vi "PreLoading.vi"(4 "Voltage":dbl=5.0 format="%#_13g", 5 "Direction":T1, 6 "target pressure [MPa]":dbl=3.0 format="%#_13g", 7 "init":bool, 8 "error in (no error)":errorcluster, 11 "Stand in":refnum<class "Stand.lvclass">) -> (0 "error out":errorcluster, 2 "done":bool, 3 "Stand out":refnum<class "Stand.lvclass">)   [LabVIEW 2019, in "Stand.lvclass"]
uses:
  Stand.lvclass
  C:/Users/ANENKOV_V1/Desktop/src/Device_class/Device.lvclass
  TypeDef/Direction.ctl
  TypeDef/SP_TYPE.ctl
  Stand.lvclass/Stand.ctl
  AI_class/AI.lvclass/AI.ctl
  AnalogComparator_class/AnalogComparator.lvclass/AnalogComparator.ctl
  Device_class/Device.lvclass/Device.ctl
  Valve Mode.ctl
  c2c3d155-81bf-490b-b50d-397c388f1e85.vi
  AnalogComparator_class/GetStatus.vi
  Valve State Mode.vi
  Valve State Mode.vi/810e184e-eeb6-4027-a8ae-1422f3ce3d45.vi
  Valve State Mode.vi/57bd4a65-f3dc-44f5-8d68-677c2a197570.vi
  Valve State Mode.vi/03b2f9e4-fceb-4725-9b90-3fd10082a088.vi
  Valve State Mode.vi/3d0d09bd-48e8-482f-b1e2-a36b2bb65234.vi
  Valve State Mode.vi/33d3f26a-dc4a-4f56-bf0a-61d04c5d7434.vi
  Valve State Mode.vi/52af9d47-24d1-4057-80bf-8d93bfb3d17d.vi
  Valve State Mode.vi/094228cb-a119-423c-9af8-5a16f059a318.vi
  Valve State Mode.vi/bf5ad1e6-a0ae-4579-ad74-ca8f304cb7cf.vi
  Valve State Mode.vi/eb4d2b76-f0f0-4e1d-bda0-609c5f37b4e7.vi
  Const All Valve.vi
  FPGA/TypeDef/DO index.ctl
  FPGA_API_class/FPGA API.lvclass
  Device_class/Device.lvclass
  AI_class/AI.lvclass
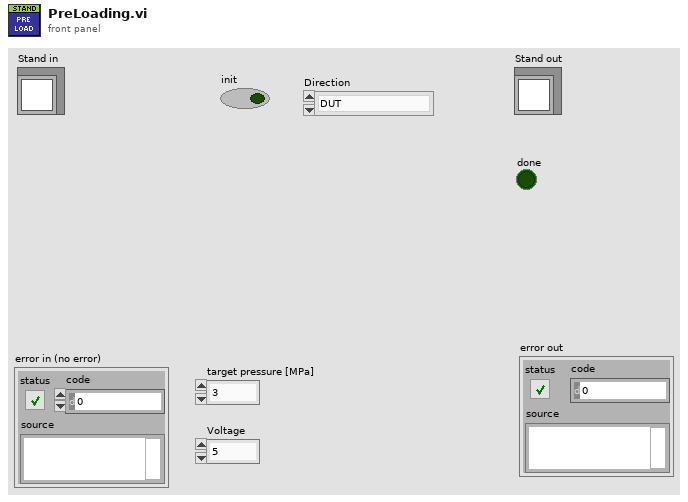
[diagram p1: front panel]
types:
  T1 = typedef "Direction.ctl" = enum8{"DUT", "Chamber"}
  T2 = typedef "SP_TYPE.ctl" = enum16{"ERROR", "ZIRO", "BASE", "SP"}
  T3 = typedef "Valve Mode.ctl" = enum16{"Filling DUT", "Filling Chamber", "Pump Pressure DUT", "Pump Pressure Chamber", "Haskel Pressure DUT", "Haskel Pressure Chamber", "Slow Release DUT", "Slow Release Chamber", "Fast Release DUT", "Fast Release Chamber", "Fast Release DUT and Chamber", "Leak Pressure DUT", "Leak Pressure Chamber", "Back Pressure DUT", "Back Pressure Chamber", "Fully Closed", "Drain", "Block DUT", "Block Chamber"}
  T4 = typedef "AI_Data.ctl" = cluster{"Stat Data":T5, "OutOfRangeMax":bool, "OutOfRangeMin":bool, "HIHI":bool, "HI":bool, "LO":bool, "LOLO":bool}
  T5 = typedef "AI Statistics Data.ctl" = cluster{"raw mean":dbl, "scl mean":dbl, "raw mean 1Hz":dbl, "scl mean 1Hz":dbl}
  T6 = typedef "DO index.ctl" = u8
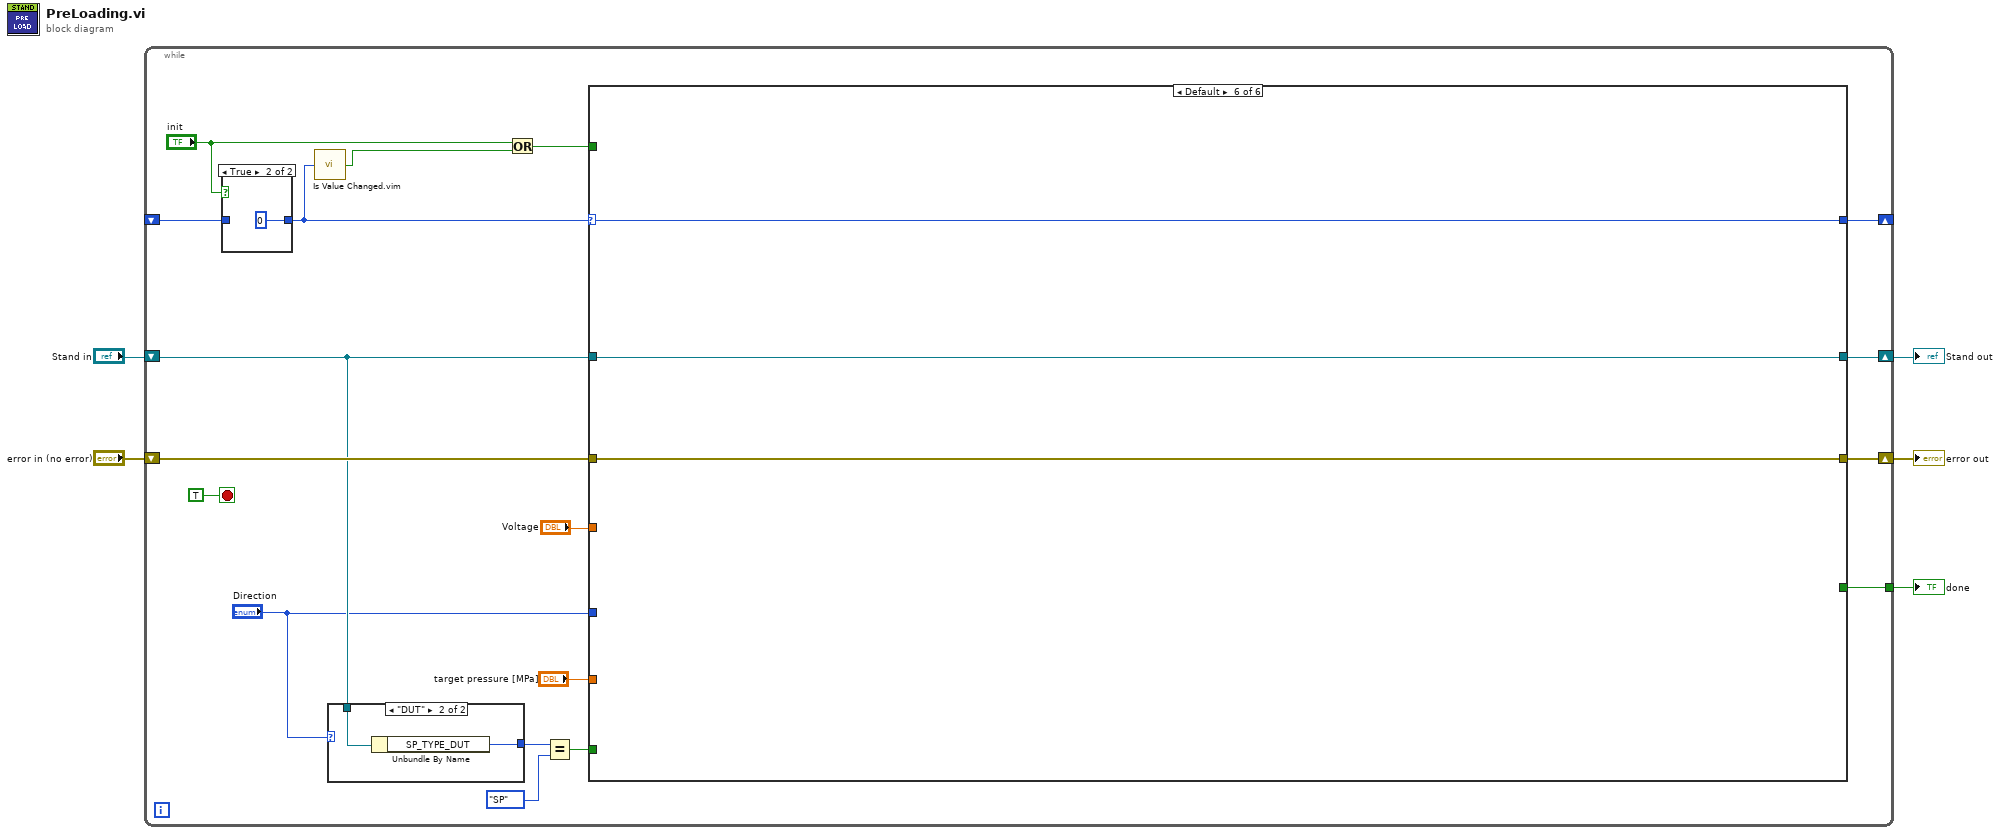
[diagram p0: block diagram]
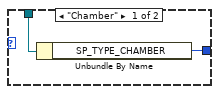
[diagram p2: hidden frame]
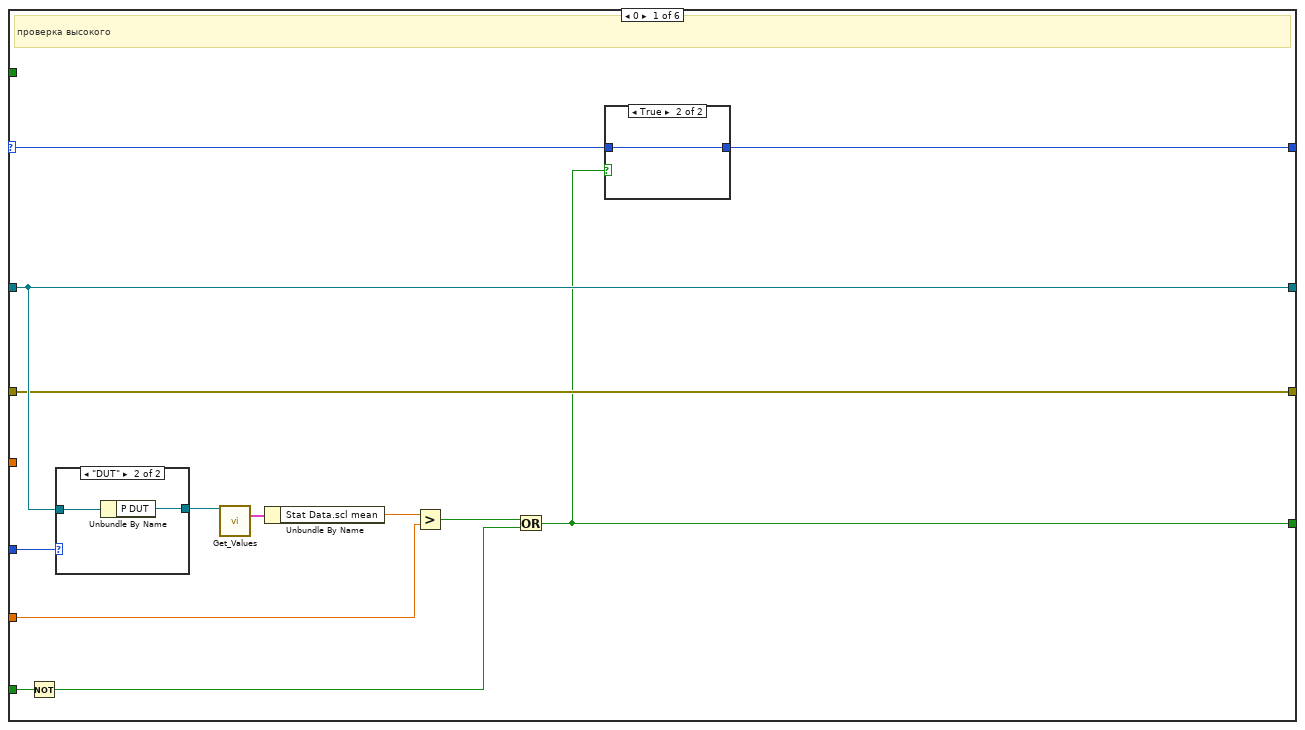
[diagram p4: hidden frame]
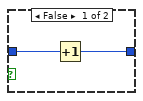
[diagram p5: hidden frame]
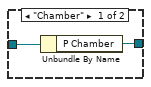
[diagram p6: hidden frame]
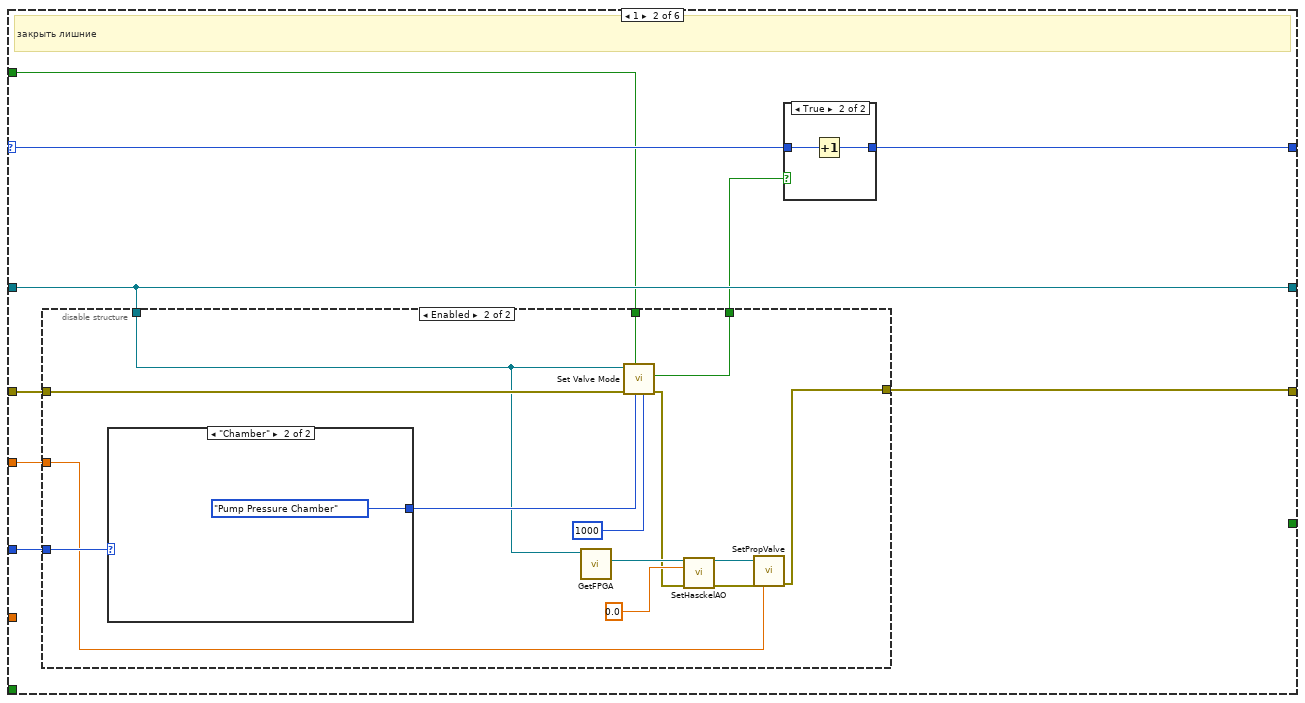
[diagram p7: hidden frame]
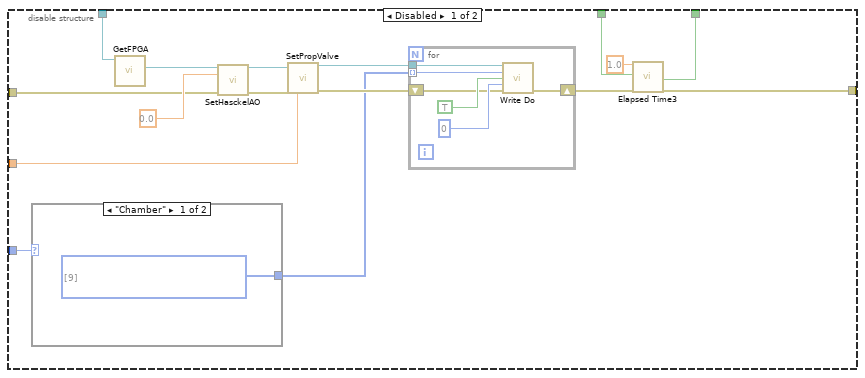
[diagram p8: hidden frame]
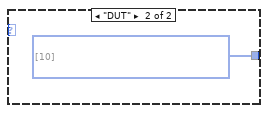
[diagram p9: hidden frame]
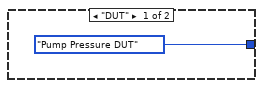
[diagram p10: hidden frame]
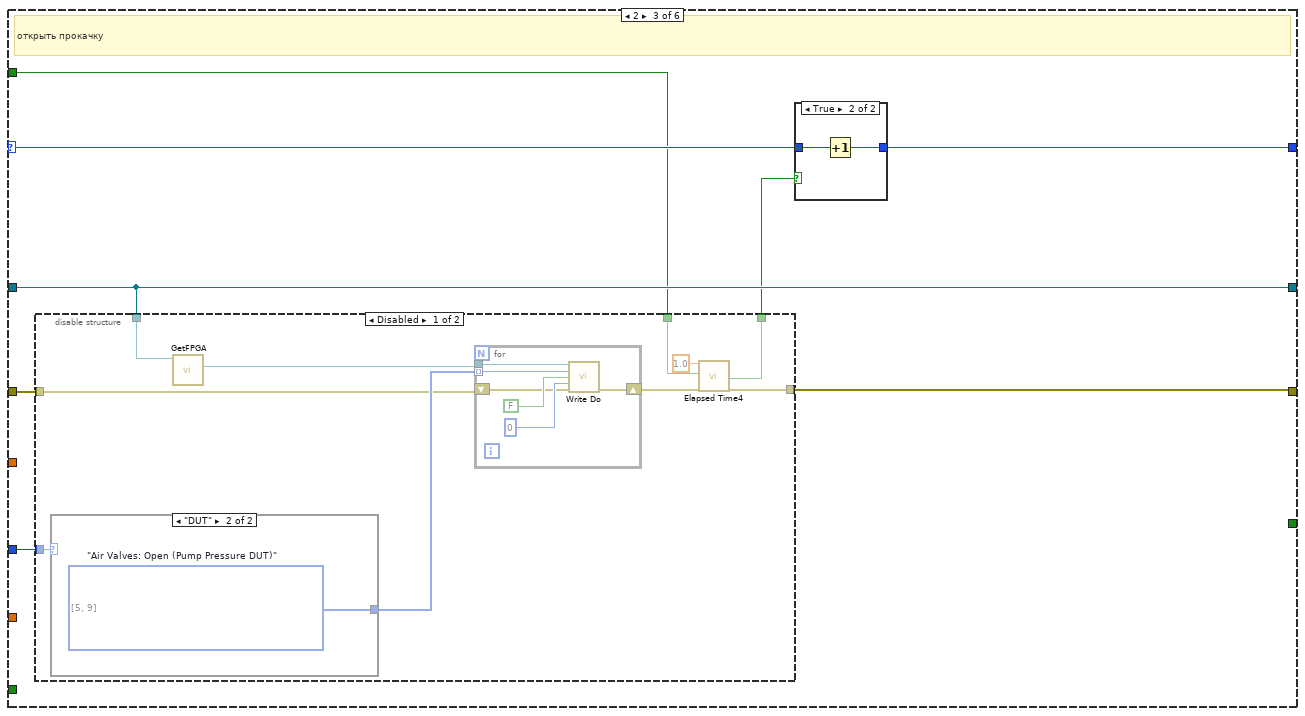
[diagram p12: hidden frame]
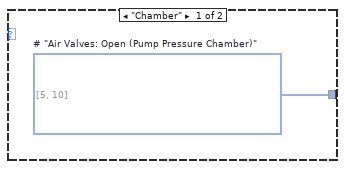
[diagram p13: hidden frame]
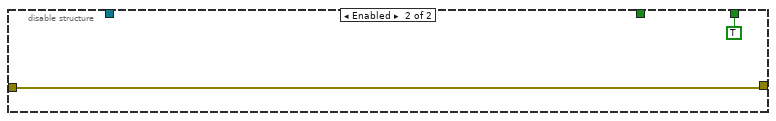
[diagram p14: hidden frame]
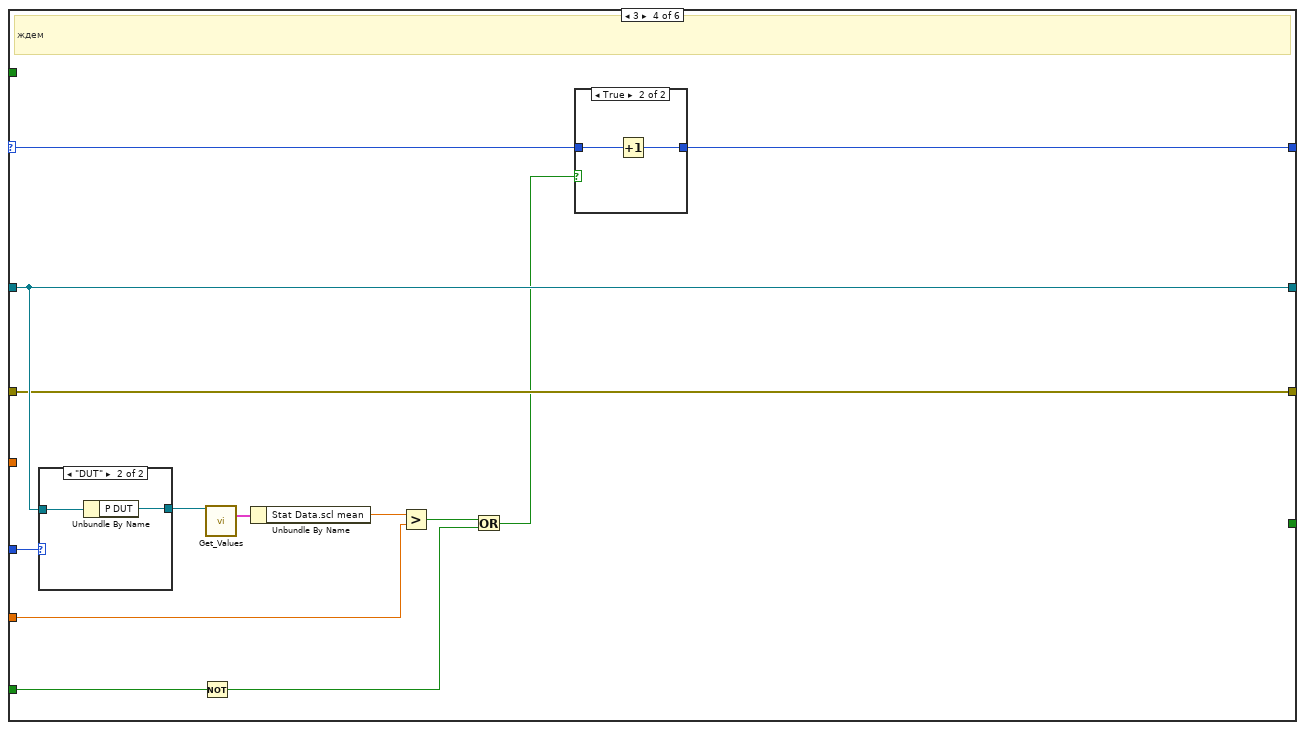
[diagram p16: hidden frame]
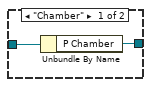
[diagram p18: hidden frame]
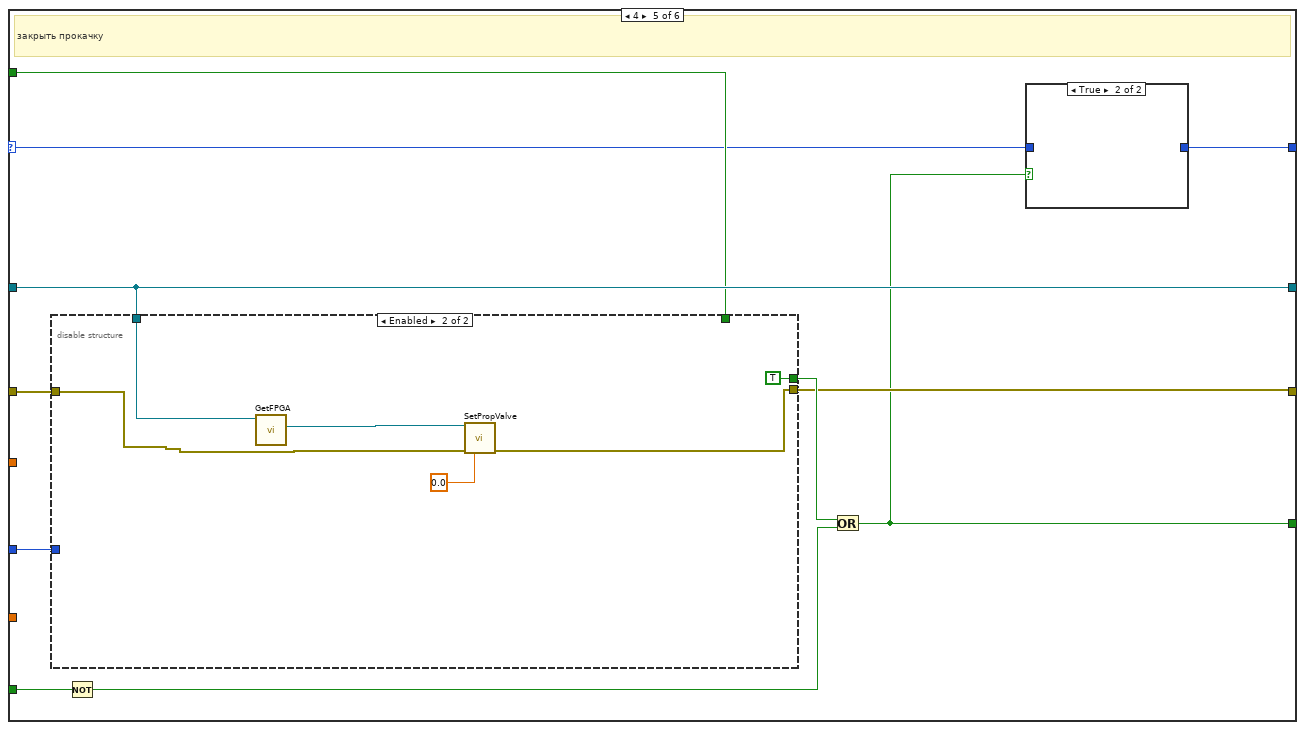
[diagram p19: hidden frame]
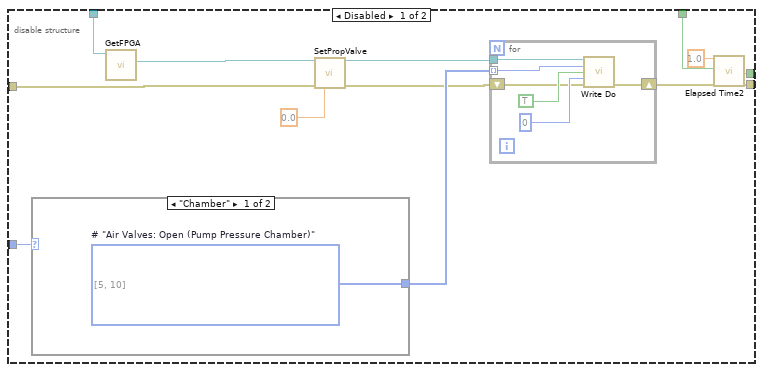
[diagram p20: hidden frame]
diagram:
  n1 = while {
    shift-right: [w21] -> _
    shift-left: _ -> [w18]
    tunnel: [w15] -> w4
    shift-right: [w14] -> w2
    shift-left: "Stand in" -> [w10]
    shift-right: [w13] -> w1
    shift-left: "error in (no error)" -> [w12]
    stop <- TRUE stop-if-true
    n2 = case shown="True" "init" {
      tunnel: w18 -> [w28 _]
      tunnel: [w28 0] -> w17
      frame False {
      }
      frame True {
      }
    }
    n3 = call "Is Value Changed.vim"("value"=w17) -> ("changed or first call?"=w22:bool)
    n4 = case shown="\"DUT\"" "Direction" {
      tunnel: w10 -> [w25 w27]
      tunnel: [w24 w26] -> w8
      frame "Chamber" {
        n5 = Unbundle By Name(w25) -> ("SP_TYPE_CHAMBER"=w24:T2)
      }
      frame "DUT" {
        n6 = Unbundle By Name(w27) -> ("SP_TYPE_DUT"=w26:T2)
      }
    }
    n7 = Or(x="init", y=w22) -> (x .or. y?=w19:bool)
    n8 = Equal?(x=w8, y=SP_TYPE."SP") -> (x = y?=w6:bool)
    n9 = case shown="Default" w17 {
      selector: w17 -> [w42 w58 w109 w145 w154 w194]
      tunnel: [w41 w57 w108 w144 w153 w194] -> w21
      tunnel: w19 -> [_ w52 w104 _ w161 _]
      tunnel: w10 -> [w34 w56 w107 w138 w163 w193]
      tunnel: "Direction" -> [w40 w53 w105 w143 w162 _]
      tunnel: "target pressure [MPa]" -> [w36 _ _ w139 _ _]
      tunnel: [w30 _ _ _ w155 _] -> w15
      tunnel: [w34 w56 w107 w138 w163 w193] -> w14
      tunnel: [w33 w50 w102 w137 w159 w192] -> w13
      tunnel: w12 -> [w33 w55 w106 w137 w158 w192]
      tunnel: "Voltage" -> [_ w54 _ _ _ _]
      tunnel: w6 -> [w32 _ _ w134 w157 _]
      frame 0 {
        # "проверка высокого"
        n10 = Not(x=w32) -> (.not. x?=w31:bool)
        n11 = case shown="\"DUT\"" w40 {
          tunnel: w34 -> [w47 w49]
          tunnel: [w46 w48] -> w37
          frame "Chamber" {
            n12 = Unbundle By Name(w47) -> ("P Chamber"=w46:refnum<class "AI.lvclass">)
          }
          frame "DUT" {
            n13 = Unbundle By Name(w49) -> ("P DUT"=w48:refnum<class "AI.lvclass">)
          }
        }
        n14 = call "Get_Values.vi"("reference in"=w37) -> ("Data"=w38:T4)  [unwired: 14 in]
        n15 = Unbundle By Name(w38) -> ("Stat Data.scl mean"=w39:dbl)
        n16 = Greater?(x=w39, y=w36) -> (0:w35:bool)
        n17 = Or(x=w35, y=w31) -> (x .or. y?=w30:bool)
        n18 = case shown="True" w30 {
          tunnel: w42 -> [w44 w45]
          tunnel: [w43 w45] -> w41
          frame False {
            n19 = Increment(x=w44) -> (x+1=w43:i32)
          }
          frame True {
          }
        }
      }
      frame 1 {
        # "закрыть лишние"
        n20 = disable-structure shown="Enabled" {
          disable-tunnel: w56 -> [w67 w86]
          disable-tunnel: w55 -> [w66 w95]
          disable-tunnel: w54 -> [w65 w85]
          disable-tunnel: w53 -> [w64 w92]
          disable-tunnel: w52 -> [w62 w96]
          disable-tunnel: [w60 w94] -> w51
          disable-tunnel: [w59 w83] -> w50
          frame Disabled {
            n21 = case shown="\"Chamber\"" w64 {
              tunnel: [w81 w82] -> w68
              frame "Chamber" {
                w81 = T6[] [9] items=["DO 0 [KP1] [M12]", "DO 1 [ON KP2] [M21]", "DO 2 [ON KP3] [M24]", "DO 3 [WATER Y18.1 [DO3]]", "DO 4 [WATER Y18.2 [DO4]]", "DO 5 [KP6 Y29.1 33.7]", "DO 6 [KP7 Y29.2 33.8]", "DO 7 [KP8 Y29.3 33.9]", "DO 8 [KP9 Y29.4  33.12]", "DO 9 [KP10 Y29.5 33.1]", "DO 10 [KP11 Y29.6 33.2]", "DO 11 [KP12 Y29.7  33.13]", "DO 12 [KP13 Y29.8  33.11]", "DO 13 [KP14 Y29.9 33.10]", "DO 14 [KP15 Y29.10  33.6]", "DO 15 [KP16 Y29.11  33.5]", "DO 16 [KP17 Y29.12  33.4]", "DO 17 [KP18 Y29.13 33.3]", "DO 18 [AIR KP19]", "DO 19 [STEP DRIVE EN KP20]", "DO 20 [KP21 Y44.1 OPEN]", "DO 21 [ KP22 Y44.1 CLOSE]", "DO 22 [ KP23 Y44.2 OPEN]", "DO 23", "DO 24 [STEP DRIVE 1]", "DO 25 [STEP DRIVE 2]"]
              }
              frame "DUT" {
                w82 = T6[] [10] items=["DO 0 [KP1] [M12]", "DO 1 [ON KP2] [M21]", "DO 2 [ON KP3] [M24]", "DO 3 [WATER Y18.1 [DO3]]", "DO 4 [WATER Y18.2 [DO4]]", "DO 5 [KP6 Y29.1 33.7]", "DO 6 [KP7 Y29.2 33.8]", "DO 7 [KP8 Y29.3 33.9]", "DO 8 [KP9 Y29.4  33.12]", "DO 9 [KP10 Y29.5 33.1]", "DO 10 [KP11 Y29.6 33.2]", "DO 11 [KP12 Y29.7  33.13]", "DO 12 [KP13 Y29.8  33.11]", "DO 13 [KP14 Y29.9 33.10]", "DO 14 [KP15 Y29.10  33.6]", "DO 15 [KP16 Y29.11  33.5]", "DO 16 [KP17 Y29.12  33.4]", "DO 17 [KP18 Y29.13 33.3]", "DO 18 [AIR KP19]", "DO 19 [STEP DRIVE EN KP20]", "DO 20 [KP21 Y44.1 OPEN]", "DO 21 [ KP22 Y44.1 CLOSE]", "DO 22 [ KP23 Y44.2 OPEN]", "DO 23", "DO 24 [STEP DRIVE 1]", "DO 25 [STEP DRIVE 2]"]
              }
            }
            n22 = call "GetFPGA.vi"("Device in"=w67) -> ("FPGA API.lvclass"=w74:refnum<class "FPGA API.lvclass">)  [unwired: 10 in]
            n23 = call-dynamic "SetHasckelAO.vi"("FPGA API in"=w74, "Haskel in"=0.0, "error in (no error)"=w66) -> ("FPGA API out"=w72:refnum<class "FPGA API.lvclass">, "error out"=w73:errorcluster)  [unwired: 11 in]
            n24 = call-dynamic "SetPropValve.vi"("FPGA API in"=w72, "error in (no error)"=w73, "AO 1"=w65) -> ("FPGA API out"=w70:refnum<class "FPGA API.lvclass">, "error out"=w69:errorcluster)  [unwired: 11 in]
            n25 = for {
              tunnel: w70 -> [w78]
              tunnel: w68 -> [w76] mode=indexing
              shift-right: [w75] -> w63
              shift-left: w69 -> [w77]
              n26 = call-dynamic "Write Do.vi"("FPGA API in"=w78, "#DO"=w76, "value"=TRUE, "Time uSec"=u32 0, "error in (no error)"=w77) -> ("error out"=w75:errorcluster)  [unwired: 9 in, 1 out]
            }
            n27 = call "Elapsed Time3"("Time Target (s)"=1.0, "Reset"=w62, "error in (no error)"=w63) -> ("Time has Elapsed"=w60:bool, "error out"=w59:errorcluster)  [unwired: 9 in, 6 out]
          }
          frame Enabled {
            n28 = case shown="\"Chamber\"" w92 {
              tunnel: [Valve_Mode."Pump Pressure DUT" ("Valve DIR") Valve_Mode."Pump Pressure Chamber" ("Valve DIR")] -> w91
              frame "DUT" {
              }
              frame "Chamber" {
              }
            }
            n29 = call "GetFPGA.vi"("Device in"=w86) -> ("FPGA API.lvclass"=w90:refnum<class "FPGA API.lvclass">)  [unwired: 10 in]
            n30 = call "Set Valve Mode.vi"("time after close"=u32 1000, "Valve DIR"=w91, "init"=w96, "error in (no error)"=w95, "Stand in"=w86) -> ("error out"=w84:errorcluster, "Done"=w94:bool)  [unwired: 5 in]
            n31 = call-dynamic "SetHasckelAO.vi"("FPGA API in"=w90, "Haskel in"=0.0, "error in (no error)"=w84) -> ("FPGA API out"=w88:refnum<class "FPGA API.lvclass">, "error out"=w89:errorcluster)  [unwired: 11 in]
            n32 = call-dynamic "SetPropValve.vi"("FPGA API in"=w88, "error in (no error)"=w89, "AO 1"=w85) -> ("error out"=w83:errorcluster)  [unwired: 11 in, 1 out]
          }
        }
        n33 = case shown="True" w51 {
          tunnel: w58 -> [w99 w101]
          tunnel: [w99 w100] -> w57
          frame False {
          }
          frame True {
            n34 = Increment(x=w101) -> (x+1=w100:i32)
          }
        }
      }
      frame 2 {
        # "открыть прокачку"
        n35 = disable-structure shown="Disabled" {
          disable-tunnel: w107 -> [w117 _]
          disable-tunnel: w106 -> [w116 w129]
          disable-tunnel: w105 -> [w115 _]
          disable-tunnel: w104 -> [w113 _]
          disable-tunnel: [w111 TRUE ("Time has Elapsed")] -> w103
          disable-tunnel: [w110 w129] -> w102
          frame Disabled {
            n36 = case shown="\"DUT\"" w115 {
              tunnel: [w126 w127] -> w118
              frame "Chamber" {
                w126 = T6[] [5, 10] items=["DO 0 [KP1] [M12]", "DO 1 [ON KP2] [M21]", "DO 2 [ON KP3] [M24]", "DO 3 [WATER Y18.1 [DO3]]", "DO 4 [WATER Y18.2 [DO4]]", "DO 5 [KP6 Y29.1 33.7]", "DO 6 [KP7 Y29.2 33.8]", "DO 7 [KP8 Y29.3 33.9]", "DO 8 [KP9 Y29.4  33.12]", "DO 9 [KP10 Y29.5 33.1]", "DO 10 [KP11 Y29.6 33.2]", "DO 11 [KP12 Y29.7  33.13]", "DO 12 [KP13 Y29.8  33.11]", "DO 13 [KP14 Y29.9 33.10]", "DO 14 [KP15 Y29.10  33.6]", "DO 15 [KP16 Y29.11  33.5]", "DO 16 [KP17 Y29.12  33.4]", "DO 17 [KP18 Y29.13 33.3]", "DO 18 [AIR KP19]", "DO 19 [STEP DRIVE EN KP20]", "DO 20 [KP21 Y44.1 OPEN]", "DO 21 [ KP22 Y44.1 CLOSE]", "DO 22 [ KP23 Y44.2 OPEN]", "DO 23", "DO 24 [STEP DRIVE 1]", "DO 25 [STEP DRIVE 2]"]  # # "Air Valves: Open (Pump Pressure Chamber)"
              }
              frame "DUT" {
                w127 = T6[] [5, 9] items=["DO 0 [KP1] [M12]", "DO 1 [ON KP2] [M21]", "DO 2 [ON KP3] [M24]", "DO 3 [WATER Y18.1 [DO3]]", "DO 4 [WATER Y18.2 [DO4]]", "DO 5 [KP6 Y29.1 33.7]", "DO 6 [KP7 Y29.2 33.8]", "DO 7 [KP8 Y29.3 33.9]", "DO 8 [KP9 Y29.4  33.12]", "DO 9 [KP10 Y29.5 33.1]", "DO 10 [KP11 Y29.6 33.2]", "DO 11 [KP12 Y29.7  33.13]", "DO 12 [KP13 Y29.8  33.11]", "DO 13 [KP14 Y29.9 33.10]", "DO 14 [KP15 Y29.10  33.6]", "DO 15 [KP16 Y29.11  33.5]", "DO 16 [KP17 Y29.12  33.4]", "DO 17 [KP18 Y29.13 33.3]", "DO 18 [AIR KP19]", "DO 19 [STEP DRIVE EN KP20]", "DO 20 [KP21 Y44.1 OPEN]", "DO 21 [ KP22 Y44.1 CLOSE]", "DO 22 [ KP23 Y44.2 OPEN]", "DO 23", "DO 24 [STEP DRIVE 1]", "DO 25 [STEP DRIVE 2]"]  # "Air Valves: Open (Pump Pressure DUT)"
              }
            }
            n37 = call "GetFPGA.vi"("Device in"=w117) -> ("FPGA API.lvclass"=w119:refnum<class "FPGA API.lvclass">)  [unwired: 10 in]
            n38 = for {
              tunnel: w119 -> [w123]
              tunnel: w118 -> [w121] mode=indexing
              shift-right: [w120] -> w114
              shift-left: w116 -> [w122]
              n39 = call-dynamic "Write Do.vi"("FPGA API in"=w123, "#DO"=w121, "value"=FALSE, "Time uSec"=u32 0, "error in (no error)"=w122) -> ("error out"=w120:errorcluster)  [unwired: 9 in, 1 out]
            }
            n40 = call "Elapsed Time4"("Time Target (s)"=1.0, "Reset"=w113, "error in (no error)"=w114) -> ("Time has Elapsed"=w111:bool, "error out"=w110:errorcluster)  [unwired: 9 in, 6 out]
          }
          frame Enabled {
          }
        }
        n41 = case shown="True" w103 {
          tunnel: w109 -> [w130 w132]
          tunnel: [w130 w131] -> w108
          frame False {
          }
          frame True {
            n42 = Increment(x=w132) -> (x+1=w131:i32)
          }
        }
      }
      frame 3 {
        # "ждем"
        n43 = case shown="\"DUT\"" w143 {
          tunnel: w138 -> [w150 w152]
          tunnel: [w149 w151] -> w140
          frame "Chamber" {
            n44 = Unbundle By Name(w150) -> ("P Chamber"=w149:refnum<class "AI.lvclass">)
          }
          frame "DUT" {
            n45 = Unbundle By Name(w152) -> ("P DUT"=w151:refnum<class "AI.lvclass">)
          }
        }
        n46 = Not(x=w134) -> (.not. x?=w133:bool)
        n47 = call "Get_Values.vi"("reference in"=w140) -> ("Data"=w141:T4)  [unwired: 14 in]
        n48 = Unbundle By Name(w141) -> ("Stat Data.scl mean"=w142:dbl)
        n49 = Greater?(x=w142, y=w139) -> (0:w136:bool)
        n50 = Or(x=w136, y=w133) -> (x .or. y?=w135:bool)
        n51 = case shown="True" w135 {
          tunnel: w145 -> [w146 w148]
          tunnel: [w146 w147] -> w144
          frame False {
          }
          frame True {
            n52 = Increment(x=w148) -> (x+1=w147:i32)
          }
        }
      }
      frame 4 {
        # "закрыть прокачку"
        n53 = disable-structure shown="Enabled" {
          disable-tunnel: w163 -> [w175 w187]
          disable-tunnel: w162 -> [w174 _]
          disable-tunnel: w161 -> [w172 _]
          disable-tunnel: [w170 TRUE ("Time has Elapsed")] -> w160
          disable-tunnel: [w169 w185] -> w159
          disable-tunnel: w158 -> [w167 w186]
          frame Disabled {
            n54 = case shown="\"Chamber\"" w174 {
              tunnel: [w183 w184] -> w176
              frame "Chamber" {
                w183 = T6[] [5, 10] items=["DO 0 [KP1] [M12]", "DO 1 [ON KP2] [M21]", "DO 2 [ON KP3] [M24]", "DO 3 [WATER Y18.1 [DO3]]", "DO 4 [WATER Y18.2 [DO4]]", "DO 5 [KP6 Y29.1 33.7]", "DO 6 [KP7 Y29.2 33.8]", "DO 7 [KP8 Y29.3 33.9]", "DO 8 [KP9 Y29.4  33.12]", "DO 9 [KP10 Y29.5 33.1]", "DO 10 [KP11 Y29.6 33.2]", "DO 11 [KP12 Y29.7  33.13]", "DO 12 [KP13 Y29.8  33.11]", "DO 13 [KP14 Y29.9 33.10]", "DO 14 [KP15 Y29.10  33.6]", "DO 15 [KP16 Y29.11  33.5]", "DO 16 [KP17 Y29.12  33.4]", "DO 17 [KP18 Y29.13 33.3]", "DO 18 [AIR KP19]", "DO 19 [STEP DRIVE EN KP20]", "DO 20 [KP21 Y44.1 OPEN]", "DO 21 [ KP22 Y44.1 CLOSE]", "DO 22 [ KP23 Y44.2 OPEN]", "DO 23", "DO 24 [STEP DRIVE 1]", "DO 25 [STEP DRIVE 2]"]  # # "Air Valves: Open (Pump Pressure Chamber)"
              }
              frame "DUT" {
                w184 = T6[] [5, 9] items=["DO 0 [KP1] [M12]", "DO 1 [ON KP2] [M21]", "DO 2 [ON KP3] [M24]", "DO 3 [WATER Y18.1 [DO3]]", "DO 4 [WATER Y18.2 [DO4]]", "DO 5 [KP6 Y29.1 33.7]", "DO 6 [KP7 Y29.2 33.8]", "DO 7 [KP8 Y29.3 33.9]", "DO 8 [KP9 Y29.4  33.12]", "DO 9 [KP10 Y29.5 33.1]", "DO 10 [KP11 Y29.6 33.2]", "DO 11 [KP12 Y29.7  33.13]", "DO 12 [KP13 Y29.8  33.11]", "DO 13 [KP14 Y29.9 33.10]", "DO 14 [KP15 Y29.10  33.6]", "DO 15 [KP16 Y29.11  33.5]", "DO 16 [KP17 Y29.12  33.4]", "DO 17 [KP18 Y29.13 33.3]", "DO 18 [AIR KP19]", "DO 19 [STEP DRIVE EN KP20]", "DO 20 [KP21 Y44.1 OPEN]", "DO 21 [ KP22 Y44.1 CLOSE]", "DO 22 [ KP23 Y44.2 OPEN]", "DO 23", "DO 24 [STEP DRIVE 1]", "DO 25 [STEP DRIVE 2]"]  # "Air Valves: Open (Pump Pressure DUT)"
              }
            }
            n55 = call "GetFPGA.vi"("Device in"=w175) -> ("FPGA API.lvclass"=w168:refnum<class "FPGA API.lvclass">)  [unwired: 10 in]
            n56 = call-dynamic "SetPropValve.vi"("FPGA API in"=w168, "error in (no error)"=w167, "AO 1"=0.0) -> ("FPGA API out"=w165:refnum<class "FPGA API.lvclass">, "error out"=w164:errorcluster)  [unwired: 11 in]
            n57 = for {
              tunnel: w165 -> [w180]
              tunnel: w176 -> [w178] mode=indexing
              shift-right: [w177] -> w173
              shift-left: w164 -> [w179]
              n58 = call-dynamic "Write Do.vi"("FPGA API in"=w180, "#DO"=w178, "value"=TRUE, "Time uSec"=u32 0, "error in (no error)"=w179) -> ("error out"=w177:errorcluster)  [unwired: 9 in, 1 out]
            }
            n59 = call "Elapsed Time2"("Time Target (s)"=1.0, "Reset"=w172, "error in (no error)"=w173) -> ("Time has Elapsed"=w170:bool, "error out"=w169:errorcluster)  [unwired: 9 in, 6 out]
          }
          frame Enabled {
            n60 = call "GetFPGA.vi"("Device in"=w187) -> ("FPGA API.lvclass"=w189:refnum<class "FPGA API.lvclass">)  [unwired: 10 in]
            n61 = call-dynamic "SetPropValve.vi"("FPGA API in"=w189, "error in (no error)"=w186, "AO 1"=0.0) -> ("error out"=w185:errorcluster)  [unwired: 11 in, 1 out]
          }
        }
        n62 = Not(x=w157) -> (.not. x?=w156:bool)
        n63 = Or(x=w160, y=w156) -> (x .or. y?=w155:bool)
        n64 = case shown="True" w155 {
          tunnel: w154 -> [w191 _]
          tunnel: [w191 _] -> w153
          frame False {
          }
          frame True {
          }
        }
      }
      frame Default {
      }
    }
  }
  "Stand out" <- w2
  "error out" <- w1
  "done" <- w4
